vi "JSON List.vi"(8 "error in (no error)":errorcluster, 10 "Root Path ([]=Root)":string[](array[string]), 11 "JSON in":string) -> (0 "error out":errorcluster, 1 "Keys/Indexes":string[](array[string]), 2 "Exists?":bool, 3 "Type":T1)   [LabVIEW 2019, in "labview_json.lvlib"]
doc: "Lists the next <b>Type</b> and <b>Keys/Indexes</b> in the <b>JSON in</b> string.\nSpecify the <b>Root Path</b> to the nested object key or array index.\n<b>Exists?</b> only returns True if the <b>Root Path</b> exists.\nCreated by: Ryan Pacini"
uses:
  labview_json.lvlib
  Element Type.ctl
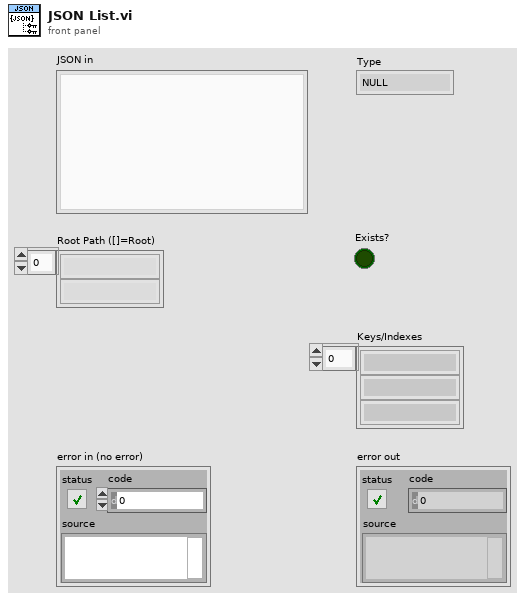
[diagram p1: front panel]
types:
  T1 = typedef "labview_json.lvlib/Element Type.ctl" = enum8{"NULL", "OBJECT", "ARRAY", "BOOL", "INT", "UINT", "FLOAT", "STRING"}
  T2 = typedef "labview_json.lvlib/Element.ctl" = cluster{"Key":string, "Type":T1, "Value":variant, "IsRootPath":bool}
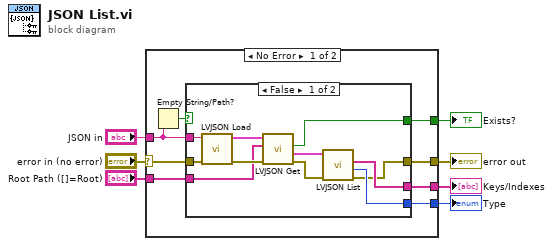
[diagram p0: block diagram]
diagram:
  n1 = case shown="No Error" "error in (no error)" {
    selector: "error in (no error)" -> [w15 w28]
    tunnel: [w10 w28] -> w6
    tunnel: "JSON in" -> [w9 _]
    tunnel: "Root Path ([]=Root)" -> [w14 _]
    tunnel: [w13 _] -> w3
    tunnel: [w12 _] -> w2
    tunnel: [w11 _] -> w1
    frame No Error {
      n2 = Empty String/Path?(string/path=w9) -> (empty?=w8:bool)
      n3 = case shown="False" w8 {
        tunnel: w15 -> [w26 w27]
        tunnel: w9 -> [w25 _]
        tunnel: w14 -> [w22 _]
        tunnel: [w21 _] -> w13
        tunnel: [w19 _] -> w12
        tunnel: [w18 _] -> w11
        tunnel: [w16 w27] -> w10
        frame False {
          n4 = call "LVJSON Load.vi"("error in (no error)"=w26, "JSON in"=w25) -> ("error out"=w24:errorcluster, "Root Element out"=w23:T2)  [unwired: 8 in]
          n5 = call "LVJSON Get.vi"("error in (no error)"=w24, "Root Path"=w22, "Root Element in"=w23) -> ("error out"=w20:errorcluster, "Element out"=w17:T2, "Exists?"=w21:bool)  [unwired: 5 in, 1 out]
          n6 = call "LVJSON List.vi"("error in (no error)"=w20, "Root Element in"=w17) -> ("error out"=w16:errorcluster, "Type"=w18:T1, "Keys/Indexes"=w19:string[])  [unwired: 6 in, 1 out]
        }
        frame True {
        }
      }
    }
    frame Error {
    }
  }
  "error out" <- w6
  "Exists?" <- w3
  "Keys/Indexes" <- w2
  "Type" <- w1
